vi "Connect.vi"(8 "error in (no error)":errorcluster, 11 "IStates in":refnum<class "IStates.lvclass">) -> (0 "error out":errorcluster, 3 "IStates out":refnum<class "IStates.lvclass">)   [LabVIEW 2023, in "HAL.lvlib" / "IScope.lvlib" / "IStates.lvclass"]
uses:
  IStates.lvclass
panel:
  out "Resource Name out":refnum<k15> caption="Session Handle out"
  in  "Resource Name":refnum<k15>
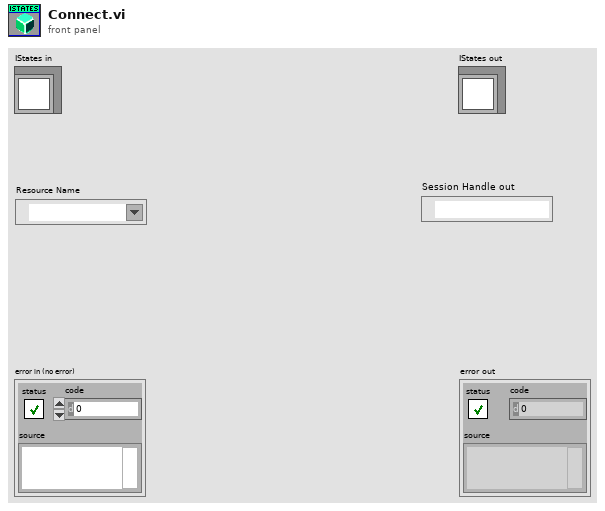
[diagram p1: front panel]
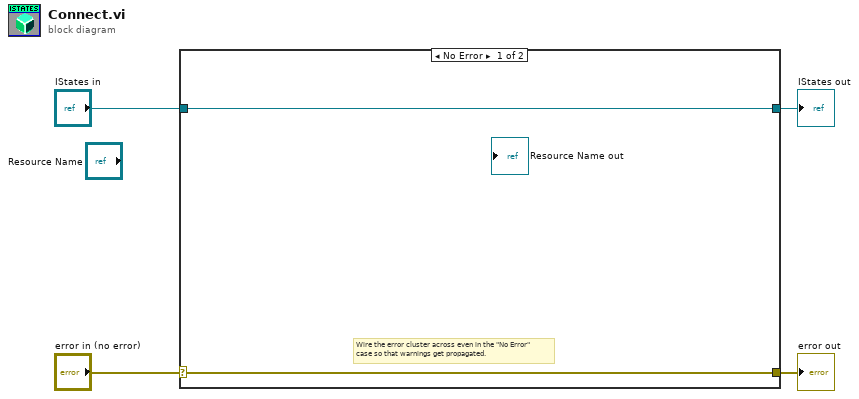
[diagram p0: block diagram]
diagram:
  n1 = case shown="No Error" "error in (no error)" {
    selector: "error in (no error)" -> [w5 w8]
    tunnel: [w5 w8] -> w3
    tunnel: [w6 w7] -> w1
    tunnel: "IStates in" -> [w6 w7]
    frame No Error {
      # "Wire the error cluster across even in the \"No Error\"\ncase so that warnings get propagated."
    }
    frame Error {
    }
  }
  "error out" <- w3
  "IStates out" <- w1
